vi "Combo box-Remap.vi"(8 "error in (no error)":errorcluster, 10 "Value":string, 11 "ComboBox in":refnum<vi>) -> (0 "error out":errorcluster)   [LabVIEW 2017]
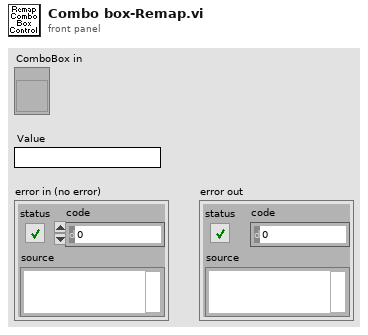
[diagram p1: front panel]
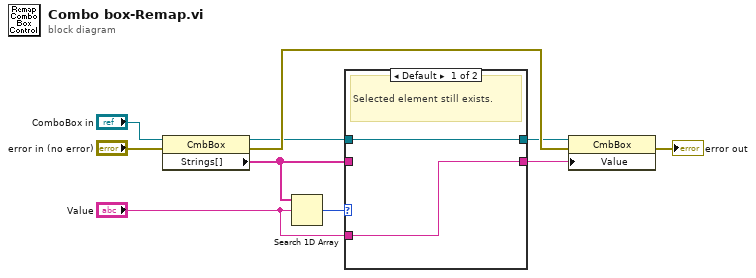
[diagram p0: block diagram]
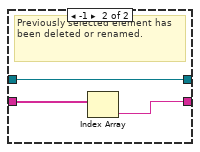
[diagram p2: hidden frame]
diagram:
  n1 = property on="Property Node" class="CmbBox"(reference="ComboBox in", error in="error in (no error)") -> (reference out=w6:refnum<vi>, error out=w8:errorcluster, "Strings[]"=w9:string[])
  n2 = Search 1D Array(1D array=w9, element="Value") -> (index of element=w4:i32)  [unwired: 1 in]
  n3 = case shown="Default" w4 {
    tunnel: [w12 w15] -> w7
    tunnel: w6 -> [w12 w15]
    tunnel: w9 -> [_ w14]
    tunnel: [w11 w13] -> w10
    tunnel: "Value" -> [w11 _]
    frame Default {
      # "Selected element still exists."
    }
    frame -1 {
      # "Previously selected element has been deleted or renamed."
      n4 = Index Array(array=w14) -> (element=w13:string)  [unwired: 1 in]
    }
  }
  n5 = property on="Property Node" class="CmbBox"(reference=w7, error in=w8, "Value"=w10) -> (error out=→"error out":errorcluster)  [unwired: 1 out]
